vi "get_component_type_name.vi"(8 "error in (no error)":errorcluster, 11 "GenericExperimentController in":refnum<class "GenericExperimentController.lvclass">) -> (0 "error out":errorcluster, 2 "component type":string, 3 "GenericExperimentController out":refnum<class "GenericExperimentController.lvclass">)   [LabVIEW 2010, in "GenericExperimentController.lvclass"]
uses:
  GenericExperimentController.lvclass
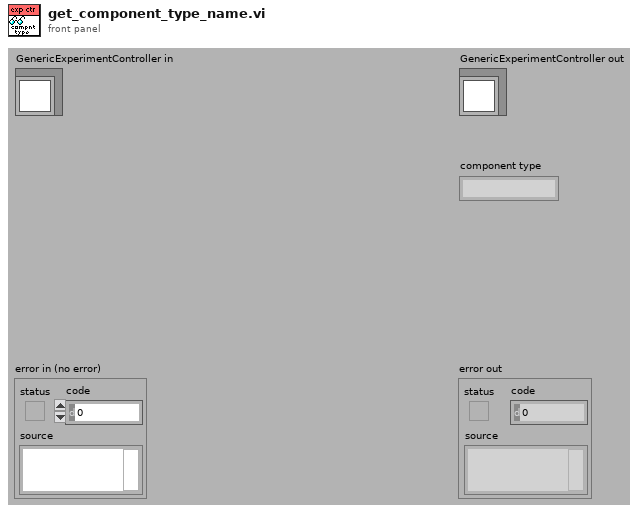
[diagram p1: front panel]
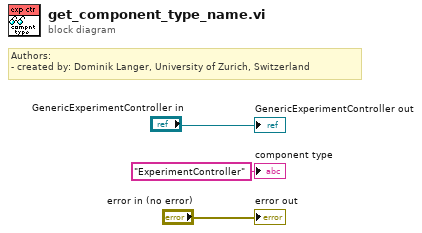
[diagram p0: block diagram]
diagram:
  # "Authors: \n- created by: Dominik Langer, University of Zurich, Switzerland"
  "error out" <- "error in (no error)"
  "GenericExperimentController out" <- "GenericExperimentController in"
  "component type" <- "ExperimentController" ("component type")
